vi "2D_Array_2_1D_Array.vi"(11 "Array in":dbl[][](array[numeric])) -> (3 "Array out":dbl[](array[numeric]))   [LabVIEW 2011]
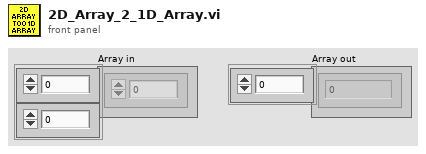
[diagram p1: front panel]
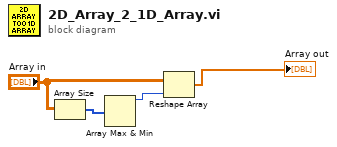
[diagram p0: block diagram]
diagram:
  n1 = Array Size(array="Array in") -> (size(s)=w2:i32[])
  n2 = Array Max & Min(array=w2) -> (max value=w3:i32)  [unwired: 3 out]
  n3 = Reshape Array("Array in", w3) -> (→"Array out":dbl[])
